vi "Setup Calibration.vi"(9 "Comm Instrument":refnum<class "Comm Instrument.lvclass">, 10 "Position":u32, 11 "Calibration in":refnum<class "Calibration.lvclass">) -> (0 "error out":errorcluster, 3 "Cree Communications out":refnum<class "Cree Communications.lvclass">)   [LabVIEW 2015, in "Calibration.lvclass"]
doc: "Setup a single position to perform calibration by creating the Comm Class and turning on Test and Cal mode."
uses:
  Calibration.lvclass
  Classes/Cree Communications/Class/Cree Communications.lvclass
  Classes/Instruments/Comm Instrument/Class/Comm Instrument.lvclass
  Classes/Cree Communications/Cree Comms Messages/Set Test Mode/Set Test Mode.lvclass
  Classes/Cree Communications/Cree Comms Messages/Write Calibration Mode/Set Calibration Mode.lvclass
  Classes/Cree Communications/Cree Comms Messages/CC Message/CC Message.lvclass/CC Message.ctl
  Classes/Cree Communications/Cree Comms Messages/CC Message/CC Message.lvclass
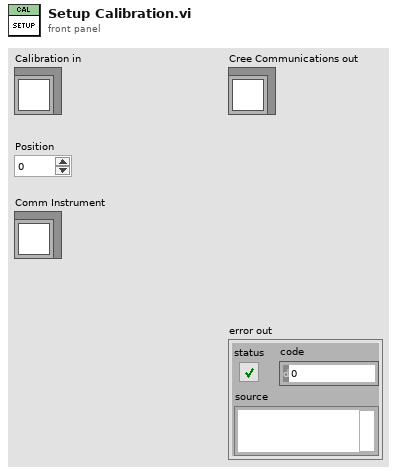
[diagram p1: front panel]
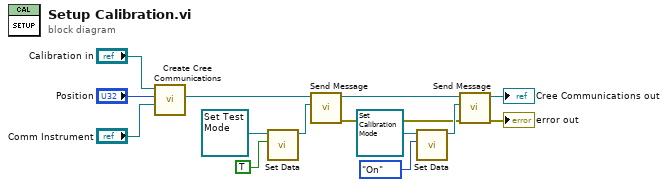
[diagram p0: block diagram]
diagram:
  n1 = call "Create Cree Communications.vi"("Comm Instrument"="Comm Instrument", "Position"="Position", "Calibration in"="Calibration in") -> ("Cree Communications"=w5:refnum<class "Cree Communications.lvclass">)  [unwired: 6 in, 2 out]
  n2 = call "Set Data.vi"("Data"=TRUE ("Message Type"), "CC Message in"=refnum<class "Set Test Mode.lvclass"> refnum ("Cree Comms Messages.lvlib:Set Test Mode.lvclass")) -> ("CC Message out"=w6:refnum<class "Set Test Mode.lvclass">)  [unwired: 8 in, 1 out]
  n3 = call "Send Message.vi"("Cree Comms Message"=w6, "Acrobat Template in"=w5) -> ("error out"=w1:errorcluster, "Acrobat Template out"=w4:refnum<class "Cree Communications.lvclass">)  [unwired: 8 in]
  n4 = call "Set Data.vi"("Data"=enum8{"Off", "On", "<Invalid>"}."On" ("Message Type"), "CC Message in"=refnum<class "Set Calibration Mode.lvclass"> refnum ("Cree Comms Messages.lvlib:Set Calibration Mode.lvclass")) -> ("CC Message out"=w7:refnum<class "Set Calibration Mode.lvclass">)  [unwired: 8 in, 1 out]
  n5 = call "Send Message.vi"("error in (no error)"=w1, "Cree Comms Message"=w7, "Acrobat Template in"=w4) -> ("error out"=→"error out":errorcluster, "Acrobat Template out"=→"Cree Communications out":refnum<class "Cree Communications.lvclass">)  [unwired: 7 in]
